vi "Configure Limit Line.vi"(7 "Limit Line Type (0: Upper)":i32(ring) items=["Upper", "Lower"], 8 "error in (no error)":errorcluster, 9 "Line Value (0 dBm)":dbl, 11 "VISA resource name":refnum<visa-resource-name>) -> (0 "error out":errorcluster, 3 "VISA resource name out":refnum<visa-resource-name>)   [LabVIEW 2022 SP3, in "Agilent N934X Series.lvlib"]
doc: "Configures Limit Lines."
uses:
  <instrlib>/Agilent N934X Series/Agilent N934X Series.lvlib
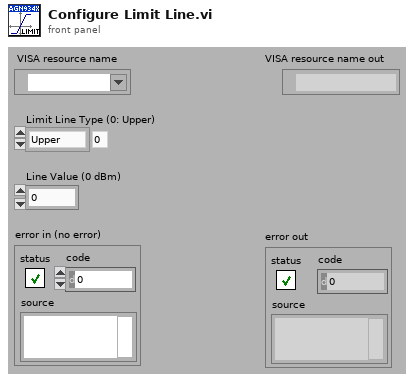
[diagram p1: front panel]
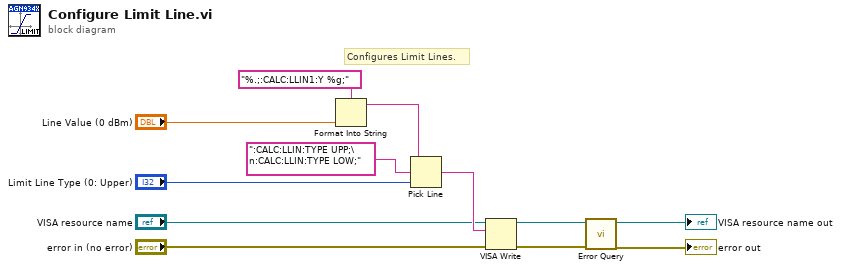
[diagram p0: block diagram]
diagram:
  # "Configures Limit Lines."
  n1 = Format Into String(format string="%.;:CALC:LLIN1:Y %g;", "Line Value (0 dBm)") -> (resulting string=w9:string)  [unwired: 2 in, 1 out]
  n2 = Pick Line(string ("")=w9, multi-line string=":CALC:LLIN:TYPE UPP;\n:CALC:LLIN:TYPE LOW;", line index="Limit Line Type (0: Upper)") -> (output string=w8:string)
  n3 = VISA Write(VISA resource name="VISA resource name", write buffer=w8, error in (no error)="error in (no error)") -> (VISA resource name out=w5:refnum<visa-resource-name>, error out=w4:errorcluster)  [unwired: 1 out]
  n4 = call <instrlib>:"Error Query.vi"("error in (no error)"=w4, "VISA resource name"=w5) -> ("error out"=→"error out":errorcluster, "VISA resource name out"=→"VISA resource name out":refnum<visa-resource-name>)  [unwired: 6 in, 2 out]
